vi "AO event parser.vi"(11 "Status":T1 {"Setting"."X Pos." scale=-5.0..5.0; "Setting"."Y Pos." scale=-5.0..5.0}) -> (3 "Stop":bool)   [LabVIEW 2013]
uses:
  init/init-status.ctl
  init/Setting.ctl
  event-package.ctl
  Event1.ctl
  data-package.ctl
  Event.ctl
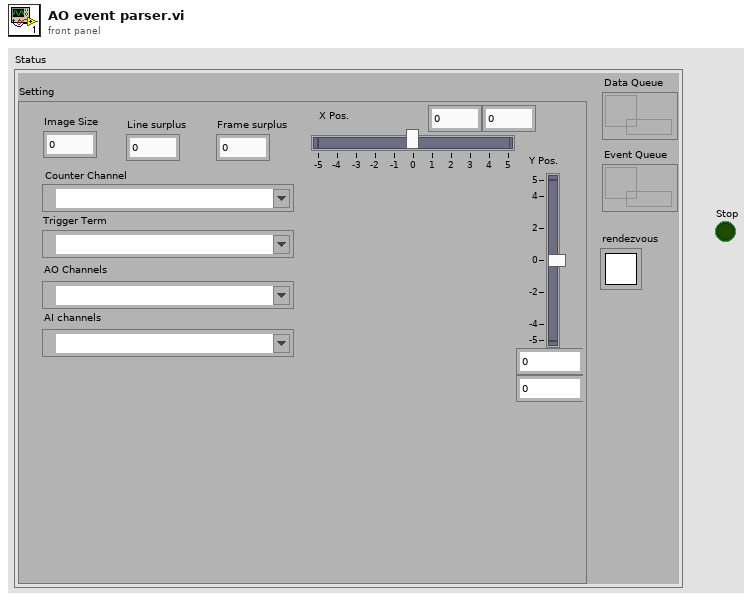
[diagram p1: front panel]
types:
  T1 = typedef "init-status.ctl" = cluster{"Setting":T2, "Event Queue":refnum<queue>, "Data Queue":refnum<queue>, "rendezvous":T3}
  T2 = typedef "Setting.ctl" = cluster{"Image Size":i32, "Counter Channel":tag, "Trigger Term":tag, "AO Channels":tag, "Y Pos.":cluster{dbl, dbl}, "X Pos.":cluster{dbl, dbl}, "Line surplus":i32, "Frame surplus":i32, "AI channels":tag}
  T3 = typedef "Rendezvous RefNum" = refnum<k1>
  T4 = typedef "event-package.ctl" = cluster{"Event":T5, "Data":string}
  T5 = typedef "Event1.ctl" = enum16{"null", "stop AI", "stop AO", "stop Counter", "save", "restart", ""}
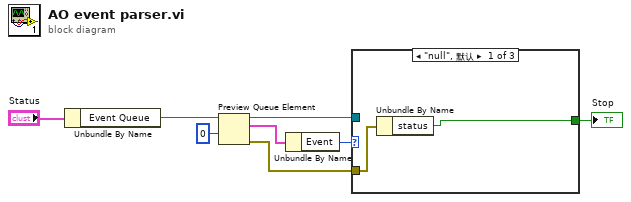
[diagram p0: block diagram]
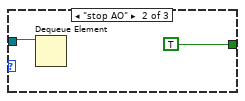
[diagram p2: hidden frame]
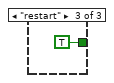
[diagram p3: hidden frame]
diagram:
  n1 = Unbundle By Name("Status") -> ("Event Queue"=w7:refnum<queue>)
  n2 = Preview Queue Element(queue=w7, timeout in ms (-1)=0 ("超时毫秒(-1)")) -> (queue out=w3:refnum<queue>, element=w6:T4, error out=w1:errorcluster)  [unwired: 1 in, 1 out]
  n3 = Unbundle By Name(w6) -> ("Event"=w4:T5)
  n4 = case shown="\"null\", 默认" w4 {
    tunnel: w3 -> [_ w12 _]
    tunnel: [w9 TRUE TRUE] -> w2
    tunnel: w1 -> [w10 _ _]
    frame "null", Default {
      n5 = Unbundle By Name(w10) -> ("status"=w9:bool)
    }
    frame "stop AO" {
      n6 = Dequeue Element(queue=w12) -> ()  [unwired: 2 in, 4 out]
    }
    frame "restart" {
    }
  }
  "Stop" <- w2
